vi "sandbox2.vi"() -> ()   [LabVIEW 2016]
panel:
  out "x .and. y?":u8
  out ".not. x?":u8 format="%b"
  out "appended array":u8[](array[numeric])
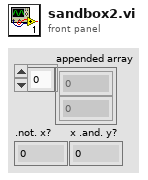
[diagram p1: front panel]
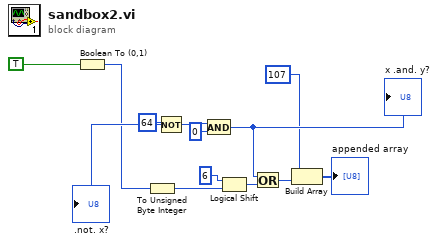
[diagram p0: block diagram]
diagram:
  n1 = Boolean To (0,1)(Boolean=TRUE ("Sleep?")) -> (0, 1=w6:i16)
  n2 = To Unsigned Byte Integer(number=w6) -> (unsigned 8bit integer=w5:u8)
  n3 = Not(x=u8 64) -> (.not. x?=w10:u8)
  ".not. x?" <- w10
  n4 = And(x=w10, y=u8 0) -> (x .and. y?=w8:u8)
  "x .and. y?" <- w8
  n5 = Logical Shift(y=u8 6 ("x"), x=w5) -> (x << y=w4:u8)
  n6 = Or(x=w8, y=w4) -> (x .or. y?=w12:u8)
  n7 = Build Array(107, w12) -> (→"appended array":i32[])
